vi "AUTON_Index.vi"(0 "Auton Array":dbl[][](array[numeric]), 5 "MeasuredHeading":dbl, 7 "LeftEncoder":dbl, 9 "RightEncoder":dbl) -> (4 "Right Drive":dbl, 6 "Left Drive":dbl, 8 "Shooter Elevation":dbl, 10 "Shooter Wheel F":dbl, 15 "Shooter Wheel B":dbl)   [LabVIEW 2012]
uses:
  Robot Global Data.vi
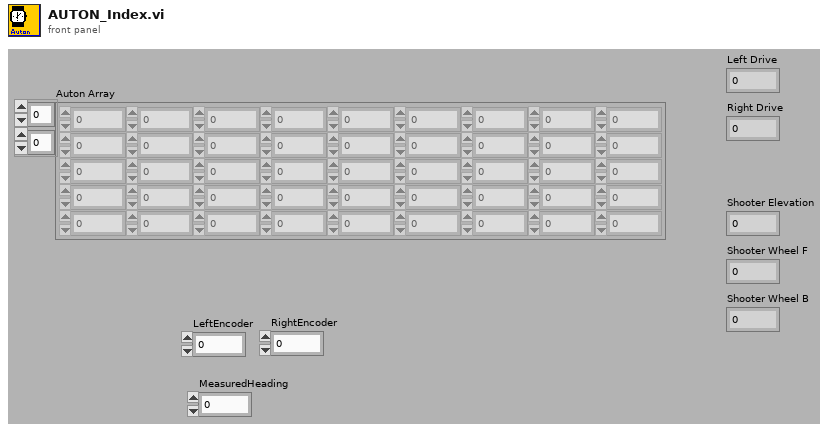
[diagram p1: front panel]
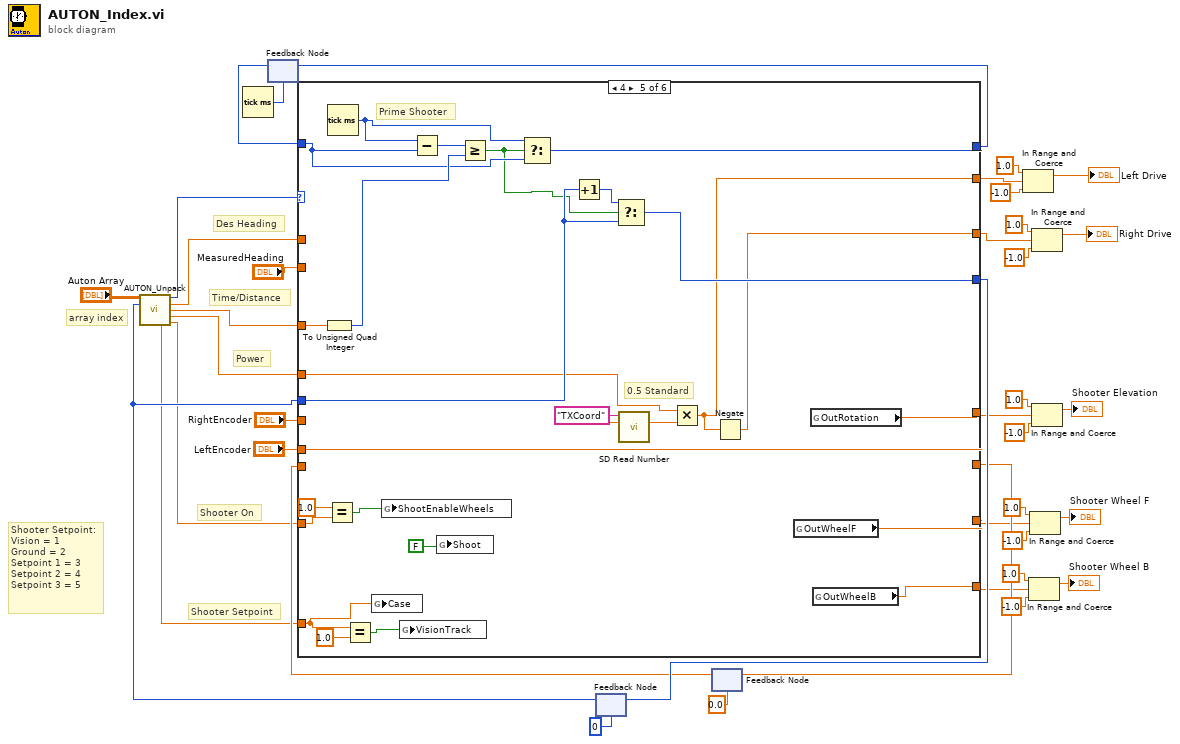
[diagram p0: block diagram]
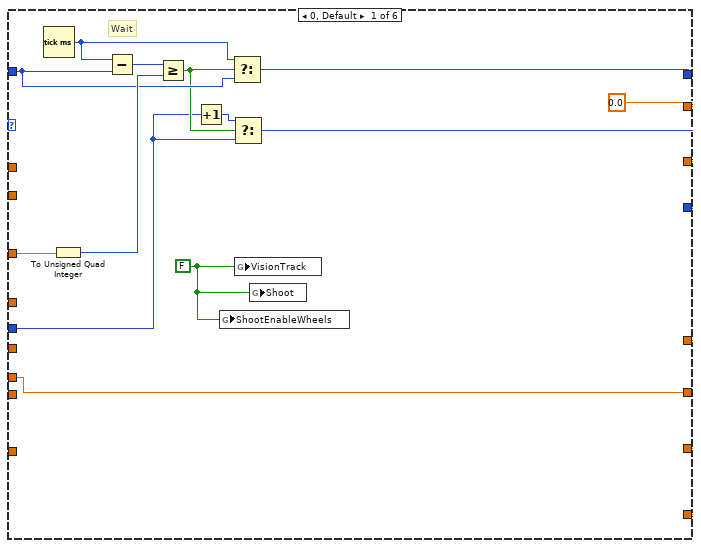
[diagram p2: hidden frame]
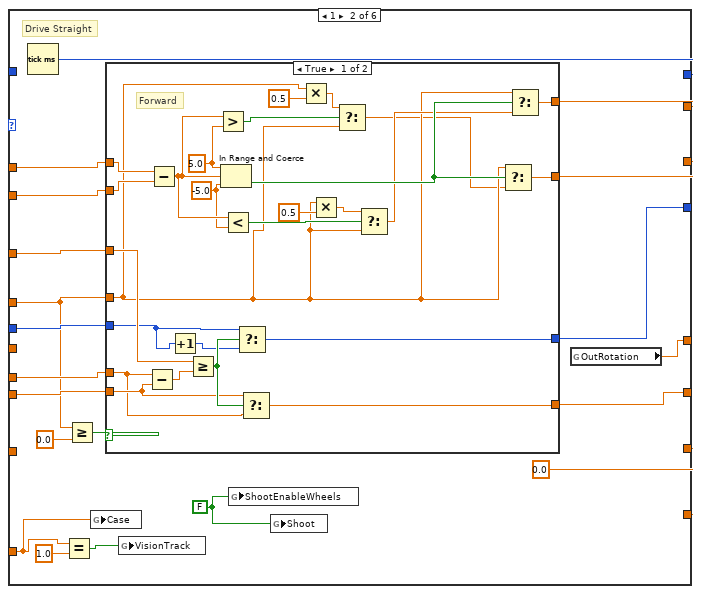
[diagram p3: hidden frame]
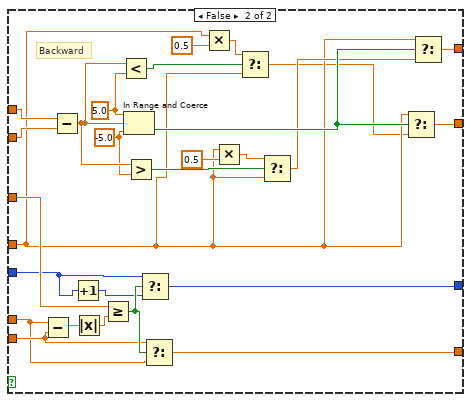
[diagram p4: hidden frame]
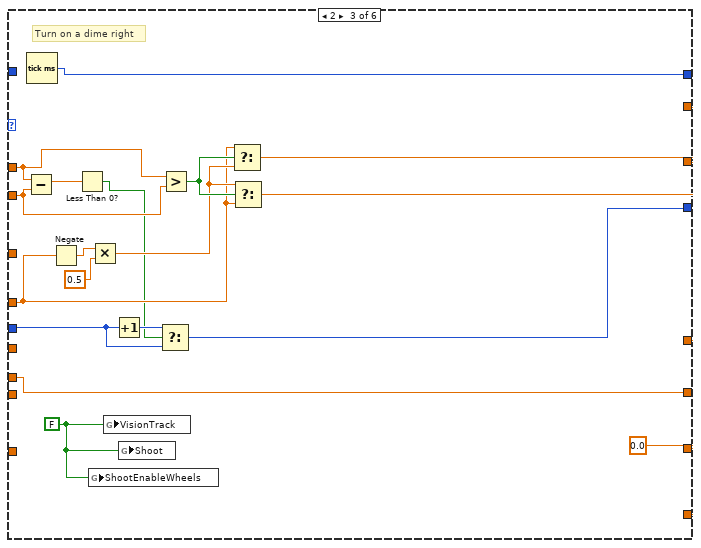
[diagram p5: hidden frame]
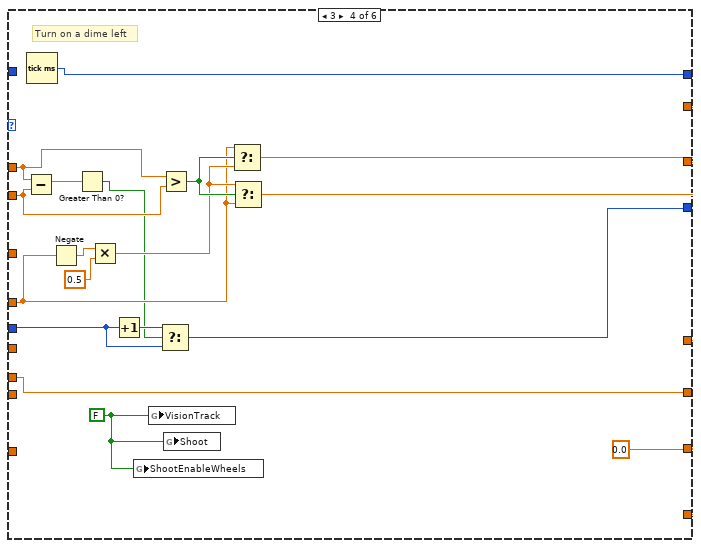
[diagram p6: hidden frame]
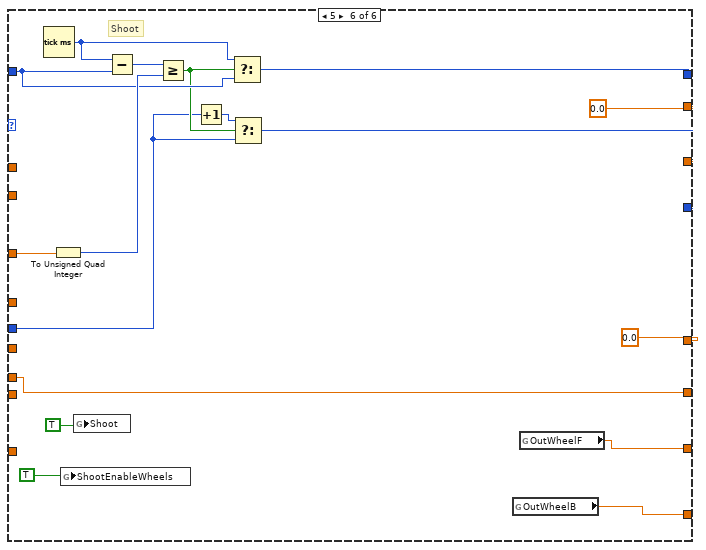
[diagram p7: hidden frame]
diagram:
  # "Shooter Setpoint:\nVision = 1\nGround = 2\nSetpoint 1 = 3\nSetpoint 2 = 4\nSetpoint 3 = 5"
  # "Shooter On"
  # "Shooter Setpoint"
  # "Des Heading"
  # "Time/Distance"
  # "Power"
  # "array index"
  n1 = Tick Count (ms)() -> (millisecond timer value=w36:u32)
  n2 = feedback #1(w36) -> (w38:u32)
  n3 = feedback #2(0) -> (w15:i32)
  n4 = call "AUTON_Unpack.vi"("all rows"="Auton Array", "Index"=w15) -> ("Primitive ID"=w19:i16, "Desired Heading"=w17:dbl, "Time/Distance"=w16:dbl, "Power"=w18:dbl, "Shooter Case"=w1:dbl, "Shooter On"=w14:dbl)  [unwired: 6 in, 2 out]
  n5 = feedback #3(0.0) -> (w21:dbl)
  n6 = case shown="4" w19 {
    tunnel: [w44 w70 w138 w156 w186 w196] -> w24
    tunnel: w15 -> [w45 w65 w141 w159 w177 w197]
    tunnel: [w52 w62 w143 w161 w175 w204] -> w26
    tunnel: w38 -> [w49 _ _ _ w176 w201]
    tunnel: w16 -> [w43 w71 _ _ w178 w195]
    tunnel: w17 -> [_ w69 w136 w154 _ _]
    tunnel: [w40 w67 w139 w157 w171 w194] -> w34
    tunnel: [w40 w66 w140 w158 w170 w194] -> w27
    tunnel: w18 -> [_ w61 w130 w148 w172 _]
    tunnel: "LeftEncoder" -> [w41 w63 w137 w155 w187 w192]
    tunnel: "MeasuredHeading" -> [_ w68 w135 w153 _ _]
    tunnel: "RightEncoder" -> [_ _ _ _ _ _]
    tunnel: w21 -> [_ w64 _ _ _ _]
    tunnel: [w41 w72 w137 w155 w187 w192] -> w20
    tunnel: w14 -> [_ _ _ _ w168 _]
    tunnel: w1 -> [_ w55 _ _ w182 _]
    tunnel: [w40 w53 w127 w144 w164 w188] -> w4
    tunnel: [w40 w53 w127 w144 w165 w189] -> w3
    tunnel: [w40 w54 w127 w144 w174 0.0 ("ShootOutElev")] -> w2
    frame 0, Default {
      w42 = FALSE ("ShootTrackEnable")
      w40 = 0.0 ("Numeric")
      # "Wait"
      n7 = Tick Count (ms)() -> (millisecond timer value=w48:u32)
      n8 = To Unsigned Quad Integer(1:w43) -> (0:w50:u64)
      n9 = Subtract(x=w48, y=w49) -> (x-y=w51:u32)
      n10 = Greater Or Equal?(x=w51, y=w50) -> (x >= y?=w47:bool)
      n11 = Increment(x=w45) -> (x+1=w46:i32)
      n12 = global write "Robot Global Data.vi" "ShootEnableWheels"(w42) -> ()
      n13 = Select(t=w48, s=w47, f=w49) -> (s? t:f=w52:u32)
      n14 = Select(t=w46, s=w47, f=w45) -> (s? t:f=w44:i32)
      n15 = global write "Robot Global Data.vi" "VisionTrack"(w42) -> ()
      n16 = global write "Robot Global Data.vi" "Shoot"(w42) -> ()
    }
    frame 1 {
      w58 = FALSE ("ShootTrackEnable")
      w53 = 0.0 ("Numeric")
      # "Drive Straight"
      n17 = Tick Count (ms)() -> (millisecond timer value=w62:u32)
      n18 = Equal?(x=w55, y=1.0) -> (x = y?=w56:bool)
      n19 = Greater Or Equal?(x=w61, y=0.0) -> (x >= y?=w59:bool)
      n20 = global write "Robot Global Data.vi" "Case"(w55) -> ()
      n21 = case shown="True" w59 {
        tunnel: [w98 w125] -> w72
        tunnel: w71 -> [w96 w124]
        tunnel: [w94 w122] -> w70
        tunnel: w69 -> [w93 w121]
        tunnel: w68 -> [w92 w120]
        tunnel: [w90 w118] -> w67
        tunnel: [w89 w117] -> w66
        tunnel: w61 -> [w78 w106]
        tunnel: w65 -> [w75 w103]
        tunnel: w64 -> [w74 w102]
        tunnel: w63 -> [w73 w101]
        frame True {
          w86 = -5.0 ("lower limit")
          w88 = 5.0 ("upper limit")
          # "Forward"
          n22 = Subtract(x=w73, y=w74) -> (x-y=w97:dbl)
          n23 = Subtract(x=w93, y=w92) -> (x-y=w87:dbl)
          n24 = Increment(x=w75) -> (x+1=w76:i32)
          n25 = Greater Or Equal?(x=w96, y=w97) -> (x >= y?=w95:bool)
          n26 = Greater?(x=w87, y=w88) -> (0:w81:bool)
          n27 = In Range and Coerce(upper limit=w88, x=w87, lower limit=w86) -> (In Range?=w91:bool)  [unwired: 1 out]
          n28 = Less?(x=w87, y=w86) -> (x < y?=w85:bool)
          n29 = Select(t=w75, s=w95, f=w76) -> (s? t:f=w94:i32)
          n30 = Select(t=w74, s=w95, f=w73) -> (s? t:f=w98:dbl)
          n31 = Multiply(x=w78, y=0.5) -> (x*y=w80:dbl)
          n32 = Multiply(x=w78, y=0.5) -> (x*y=w83:dbl)
          n33 = Select(t=w80, s=w81, f=w78) -> (s? t:f=w77:dbl)
          n34 = Select(t=w83, s=w85, f=w78) -> (s? t:f=w82:dbl)
          n35 = Select(t=w78, s=w91, f=w77) -> (s? t:f=w89:dbl)
          n36 = Select(t=w78, s=w91, f=w82) -> (s? t:f=w90:dbl)
        }
        frame False {
          w114 = -5.0 ("lower limit")
          w116 = 5.0 ("upper limit")
          # "Backward"
          n37 = Subtract(x=w101, y=w102) -> (x-y=w99:dbl)
          n38 = Subtract(x=w121, y=w120) -> (x-y=w115:dbl)
          n39 = Increment(x=w103) -> (x+1=w104:i32)
          n40 = Absolute Value(x=w99) -> (abs(x)=w100:dbl)
          n41 = Greater Or Equal?(x=w124, y=w100) -> (x >= y?=w123:bool)
          n42 = Less?(x=w115, y=w116) -> (x < y?=w109:bool)
          n43 = In Range and Coerce(upper limit=w116, x=w115, lower limit=w114) -> (In Range?=w119:bool)  [unwired: 1 out]
          n44 = Greater?(x=w115, y=w114) -> (0:w113:bool)
          n45 = Select(t=w103, s=w123, f=w104) -> (s? t:f=w122:i32)
          n46 = Select(t=w102, s=w123, f=w101) -> (s? t:f=w125:dbl)
          n47 = Multiply(x=w106, y=0.5) -> (x*y=w108:dbl)
          n48 = Multiply(x=w106, y=0.5) -> (x*y=w111:dbl)
          n49 = Select(t=w108, s=w109, f=w106) -> (s? t:f=w105:dbl)
          n50 = Select(t=w111, s=w113, f=w106) -> (s? t:f=w110:dbl)
          n51 = Select(t=w106, s=w119, f=w105) -> (s? t:f=w117:dbl)
          n52 = Select(t=w106, s=w119, f=w110) -> (s? t:f=w118:dbl)
        }
      }
      n53 = global write "Robot Global Data.vi" "VisionTrack"(w56) -> ()
      n54 = global write "Robot Global Data.vi" "ShootEnableWheels"(w58) -> ()
      n55 = global write "Robot Global Data.vi" "Shoot"(w58) -> ()
      n56 = global read "Robot Global Data.vi" "OutRotation"() -> (w54:dbl)
    }
    frame 2 {
      w126 = FALSE ("ShootTrackEnable")
      w127 = 0.0 ("Numeric")
      # "Turn on a dime right"
      n57 = Subtract(x=w136, y=w135) -> (x-y=w129:dbl)
      n58 = Tick Count (ms)() -> (millisecond timer value=w143:u32)
      n59 = Negate(x=w130) -> (-x=w133:dbl)
      n60 = Less Than 0?(x=w129) -> (x < 0?=w128:bool)
      n61 = global write "Robot Global Data.vi" "ShootEnableWheels"(w126) -> ()
      n62 = Multiply(x=w133, y=0.5) -> (x*y=w131:dbl)
      n63 = global write "Robot Global Data.vi" "VisionTrack"(w126) -> ()
      n64 = Increment(x=w141) -> (x+1=w142:i32)
      n65 = global write "Robot Global Data.vi" "Shoot"(w126) -> ()
      n66 = Select(t=w142, s=w128, f=w141) -> (s? t:f=w138:i32)
      n67 = Greater?(x=w136, y=w135) -> (0:w134:bool)
      n68 = Select(t=w130, s=w134, f=w131) -> (s? t:f=w139:dbl)
      n69 = Select(t=w131, s=w134, f=w130) -> (s? t:f=w140:dbl)
    }
    frame 3 {
      w145 = FALSE ("ShootTrackEnable")
      w144 = 0.0 ("Numeric")
      # "Turn on a dime left"
      n70 = Subtract(x=w154, y=w153) -> (x-y=w147:dbl)
      n71 = Tick Count (ms)() -> (millisecond timer value=w161:u32)
      n72 = Negate(x=w148) -> (-x=w151:dbl)
      n73 = Greater Than 0?(x=w147) -> (x > 0?=w146:bool)
      n74 = Multiply(x=w151, y=0.5) -> (x*y=w149:dbl)
      n75 = Increment(x=w159) -> (x+1=w160:i32)
      n76 = global write "Robot Global Data.vi" "ShootEnableWheels"(w145) -> ()
      n77 = global write "Robot Global Data.vi" "VisionTrack"(w145) -> ()
      n78 = Select(t=w160, s=w146, f=w159) -> (s? t:f=w156:i32)
      n79 = Greater?(x=w154, y=w153) -> (0:w152:bool)
      n80 = global write "Robot Global Data.vi" "Shoot"(w145) -> ()
      n81 = Select(t=w148, s=w152, f=w149) -> (s? t:f=w157:dbl)
      n82 = Select(t=w149, s=w152, f=w148) -> (s? t:f=w158:dbl)
    }
    frame 4 {
      # "0.5 Standard"
      # "Prime Shooter"
      n83 = To Unsigned Quad Integer(1:w178) -> (0:w180:u64)
      n84 = Equal?(x=1.0, y=w168) -> (x = y?=w166:bool)
      n85 = Tick Count (ms)() -> (millisecond timer value=w179:u32)
      n86 = Equal?(x=w182, y=1.0) -> (x = y?=w183:bool)
      n87 = global write "Robot Global Data.vi" "Case"(w182) -> ()
      n88 = global write "Robot Global Data.vi" "ShootEnableWheels"(w166) -> ()
      n89 = global write "Robot Global Data.vi" "VisionTrack"(w183) -> ()
      n90 = Subtract(x=w179, y=w176) -> (x-y=w181:u32)
      n91 = global write "Robot Global Data.vi" "Shoot"(FALSE ("Shoot")) -> ()
      n92 = Greater Or Equal?(x=w181, y=w180) -> (x >= y?=w173:bool)
      n93 = Select(t=w179, s=w173, f=w176) -> (s? t:f=w175:u32)
      n94 = Increment(x=w177) -> (x+1=w185:i32)
      n95 = Select(t=w185, s=w173, f=w177) -> (s? t:f=w186:i32)
      n96 = call <vilib>:"SD Read Number.vi"("Name"="TXCoord") -> ("Numeric"=w162:dbl)  [unwired: 8 in, 2 out]
      n97 = Multiply(x=w172, y=w162) -> (x*y=w171:dbl)
      n98 = Negate(x=w171) -> (-x=w170:dbl)
      n99 = global read "Robot Global Data.vi" "OutWheelF"() -> (w165:dbl)
      n100 = global read "Robot Global Data.vi" "OutRotation"() -> (w174:dbl)
      n101 = global read "Robot Global Data.vi" "OutWheelB"() -> (w164:dbl)
    }
    frame 5 {
      w194 = 0.0 ("Numeric")
      # "Shoot"
      n102 = Tick Count (ms)() -> (millisecond timer value=w200:u32)
      n103 = To Unsigned Quad Integer(1:w195) -> (0:w202:u64)
      n104 = global write "Robot Global Data.vi" "ShootEnableWheels"(TRUE ("ShootEnableWheels")) -> ()
      n105 = global write "Robot Global Data.vi" "Shoot"(TRUE ("Shoot")) -> ()
      n106 = Subtract(x=w200, y=w201) -> (x-y=w203:u32)
      n107 = Greater Or Equal?(x=w203, y=w202) -> (x >= y?=w199:bool)
      n108 = Increment(x=w197) -> (x+1=w198:i32)
      n109 = Select(t=w200, s=w199, f=w201) -> (s? t:f=w204:u32)
      n110 = Select(t=w198, s=w199, f=w197) -> (s? t:f=w196:i32)
      n111 = global read "Robot Global Data.vi" "OutWheelB"() -> (w188:dbl)
      n112 = global read "Robot Global Data.vi" "OutWheelF"() -> (w189:dbl)
    }
  }
  n113 = feedback-in #1(w26) -> ()
  n114 = feedback-in #2(w24) -> ()
  n115 = feedback-in #3(w20) -> ()
  n116 = In Range and Coerce(upper limit=1.0, x=w34, lower limit=-1.0) -> (coerced(x)=→"Left Drive":dbl)  [unwired: 1 out]
  n117 = In Range and Coerce(upper limit=1.0, x=w4, lower limit=-1.0) -> (coerced(x)=→"Shooter Wheel B":dbl)  [unwired: 1 out]
  n118 = In Range and Coerce(upper limit=1.0, x=w3, lower limit=-1.0) -> (coerced(x)=→"Shooter Wheel F":dbl)  [unwired: 1 out]
  n119 = In Range and Coerce(upper limit=1.0, x=w27, lower limit=-1.0) -> (coerced(x)=→"Right Drive":dbl)  [unwired: 1 out]
  n120 = In Range and Coerce(upper limit=1.0, x=w2, lower limit=-1.0) -> (coerced(x)=→"Shooter Elevation":dbl)  [unwired: 1 out]
